vi "Delete DVR.vi"(8 "Error In":errorcluster, 11 "Data Type DVR Refs":T1[](array[typedef])) -> (0 "Error Out":errorcluster)   [LabVIEW 2023, in "Data.lvclass"]
doc: "This method deletes the data value references of the data class."
uses:
  Data.lvclass
  Controls/Data Class Details.ctl
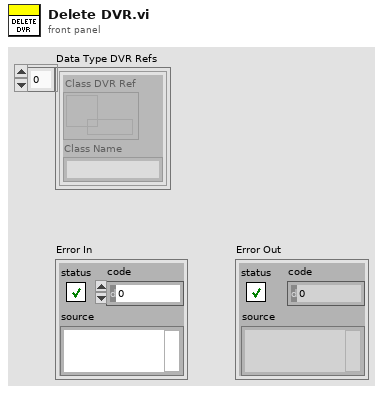
[diagram p1: front panel]
types:
  T1 = typedef "Data Class Details.ctl" = cluster{"Class DVR Ref":refnum<data-value>, "Class Name":string}
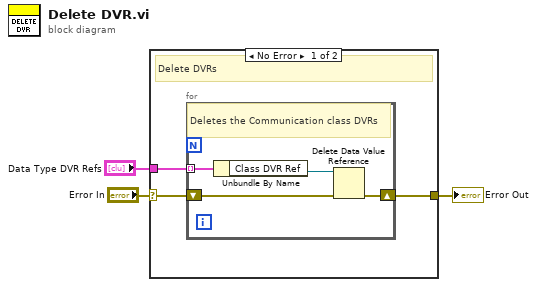
[diagram p0: block diagram]
diagram:
  n1 = case shown="No Error" "Error In" {
    selector: "Error In" -> [w6 w11]
    tunnel: [w5 w11] -> w2
    tunnel: "Data Type DVR Refs" -> [w4 _]
    frame No Error {
      # "Delete DVRs"
      n2 = for {
        shift-right: [w9] -> w5
        shift-left: w6 -> [w10]
        tunnel: w4 -> [w8] mode=indexing
        # "Deletes the Communication class DVRs"
        n3 = Unbundle By Name(w8) -> ("Class DVR Ref"=w7:refnum<data-value>)
        n4 = Delete Data Value Reference(data value reference=w7, error in=w10) -> (error out=w9:errorcluster)  [unwired: 1 out]
      }
    }
    frame Error {
    }
  }
  "Error Out" <- w2
